vi "Acquire Data.vi"(8 "error in (no error)":errorcluster, 9 "Data Queue":refnum<queue>, 10 "Data Notifier":refnum<notifier>, 11 "VISA resource name":refnum<visa-resource-name>) -> (0 "error out":errorcluster, 3 "VISA resource name out":refnum<visa-resource-name>)   [LabVIEW 2020, in "Acquisition.lvlib"]
uses:
  Acquisition.lvlib
panel:
  in  "Meas Out":T1
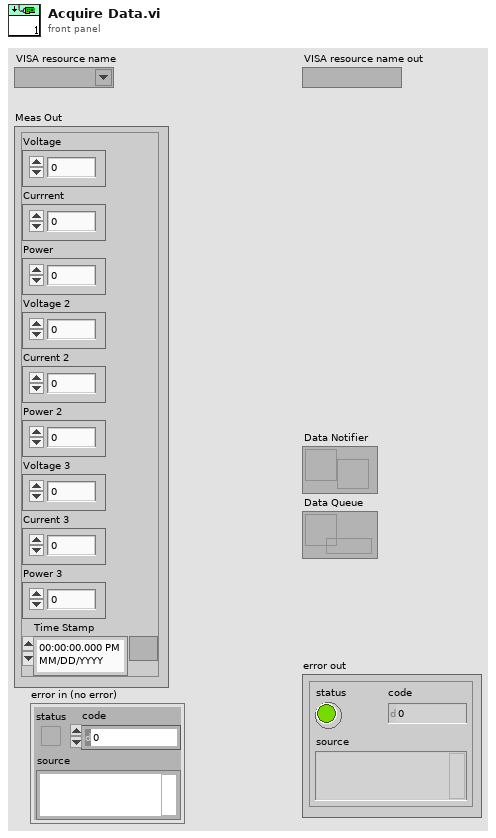
[diagram p1: front panel]
types:
  T1 = cluster{"Time Stamp":timestamp, "Voltage 3":dbl, "Voltage 2":dbl, "Voltage":dbl, "Current 3":dbl, "Current 2":dbl, "Currrent":dbl, "Power 3":dbl, "Power 2":dbl, "Power":dbl}
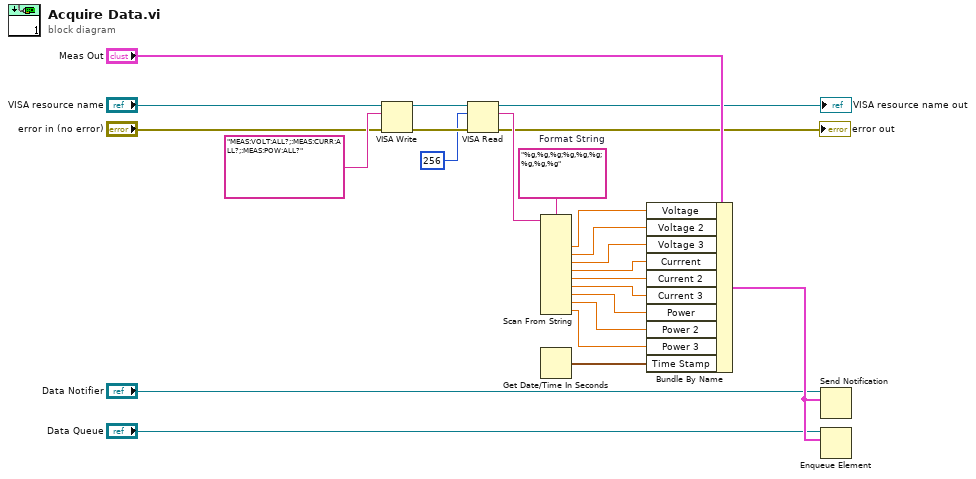
[diagram p0: block diagram]
diagram:
  w20 = "%g,%g,%g;%g,%g,%g;%g,%g,%g"  # Format String
  n1 = VISA Write(VISA resource name="VISA resource name", write buffer="MEAS:VOLT:ALL?;:MEAS:CURR:ALL?;:MEAS:POW:ALL?", error in (no error)="error in (no error)") -> (VISA resource name out=w22:refnum<visa-resource-name>, error out=w24:errorcluster)  [unwired: 1 out]
  n2 = VISA Read(VISA resource name=w22, byte count=u32 256, error in (no error)=w24) -> (VISA resource name out=→"VISA resource name out":refnum<visa-resource-name>, read buffer=w19:string, error out=→"error out":errorcluster)  [unwired: 1 out]
  n3 = Scan From String(format string=w20, input string=w19) -> (output 1=w16:dbl, output 2=w15:dbl, output 3=w8:dbl, output 4=w9:dbl, output 5=w10:dbl, output 6=w11:dbl, output 7=w12:dbl, output 8=w13:dbl, output 9=w14:dbl)  [unwired: 11 in, 3 out]
  n4 = Get Date/Time In Seconds() -> (seconds since 1Jan1904=w17:timestamp)
  n5 = Bundle By Name(cluster="Meas Out", "Voltage"=w16, "Voltage 2"=w15, "Voltage 3"=w8, "Currrent"=w9, "Current 2"=w10, "Current 3"=w11, "Power"=w12, "Power 2"=w13, "Power 3"=w14, "Time Stamp"=w17) -> (w18:T1)
  n6 = Send Notification(notification=w18, notifier="Data Notifier") -> ()  [unwired: 1 in, 2 out]
  n7 = Enqueue Element(queue="Data Queue", element=w18) -> ()  [unwired: 2 in, 3 out]
